vi "normVect.vi"(11 "Array":dbl[](array[numeric])) -> (3 "norm":dbl)   [LabVIEW 2013, in "3 dot tracker.lvlib"]
uses:
  3 dot tracker.lvlib
panel:
  # "R = sqrt(a^2 + b^2 + c^2)"
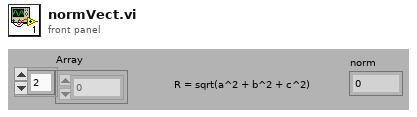
[diagram p1: front panel]
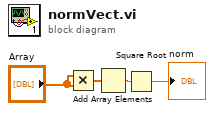
[diagram p0: block diagram]
diagram:
  n1 = Multiply(x="Array", y="Array") -> (x*y=w2:dbl[])
  n2 = Add Array Elements(numeric array=w2) -> (sum=w1:dbl)
  n3 = Square Root(x=w1) -> (sqrt(x)=→"norm":dbl)
